vi "Add BuildSpec.vi"(8 "error in (no error)":errorcluster, 10 "Build Spec Parameters":T1, 11 "Project Sync Tools in":refnum<class "Project Sync Tools.lvclass">) -> (0 "error out":errorcluster, 3 "Project Sync Tools out":refnum<class "Project Sync Tools.lvclass">)   [LabVIEW 2019, in "Project Sync Tools.lvclass"]
uses:
  Project Sync Tools.lvclass
  TypeDefs/BuildSpec Raw Parameters.ctl
  Project Sync Tools.lvclass/Project Sync Tools.ctl
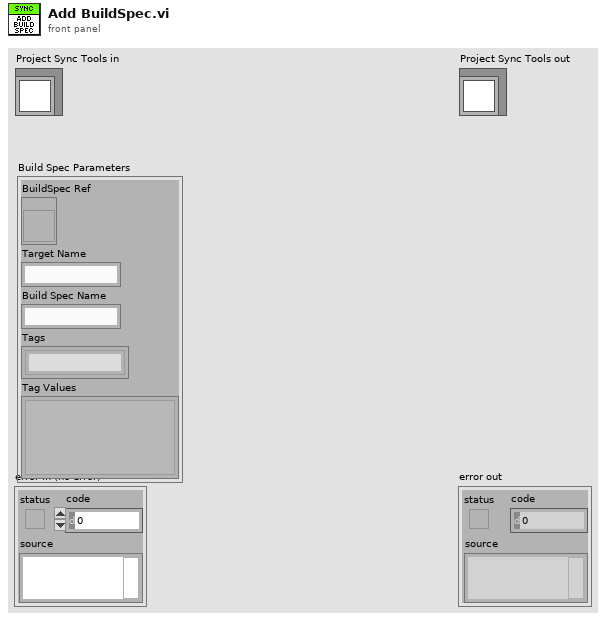
[diagram p1: front panel]
types:
  T1 = typedef "Project Sync Tools.lvclass/BuildSpec Raw Parameters.ctl" = cluster{"BuildSpec Ref":refnum<vi>, "Target Name":string, "Build Spec Name":string, "Tags":string[], "Tag Values":variant[]}
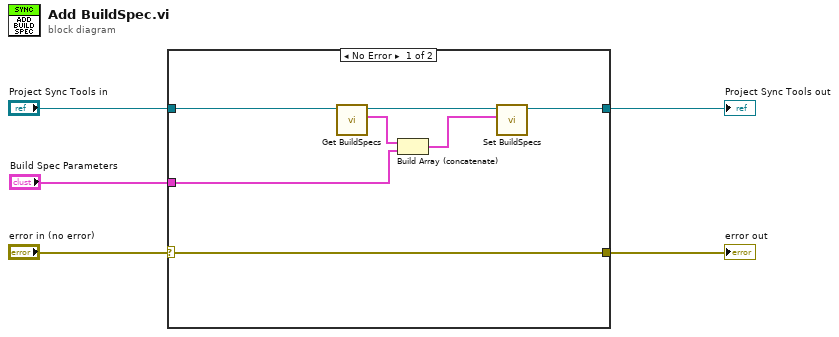
[diagram p0: block diagram]
diagram:
  n1 = case shown="No Error" "error in (no error)" {
    selector: "error in (no error)" -> [w12 w14]
    tunnel: [w12 w14] -> w4
    tunnel: [w6 w13] -> w2
    tunnel: "Project Sync Tools in" -> [w11 w13]
    tunnel: "Build Spec Parameters" -> [w9 _]
    frame No Error {
      n2 = call "Get BuildSpecs.vi"("Project Sync Tools in"=w11) -> ("BuildSpecs"=w10:T1[], "Project Sync Tools out"=w8:refnum<class "Project Sync Tools.lvclass">)  [unwired: 9 in]
      n3 = Build Array (concatenate)(w10, w9) -> (w7:T1[])
      n4 = call "Set BuildSpecs.vi"("BuildSpecs"=w7, "Project Sync Tools in"=w8) -> ("Project Sync Tools out"=w6:refnum<class "Project Sync Tools.lvclass">)  [unwired: 9 in]
    }
    frame Error {
    }
  }
  "error out" <- w4
  "Project Sync Tools out" <- w2
